vi "Global - Rendezvous.vi"() -> ()   [LabVIEW 2019]
panel:
  out "rendezvous":T1
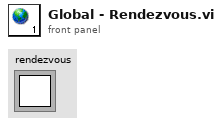
[diagram p1: front panel]
types:
  T1 = typedef "Rendezvous RefNum" = refnum<k1>
diagram:
